vi "Global Mapper H.vi"(0 "GIC Input":T1={"     Use ?\nOff       On"=[FALSE, TRUE, FALSE, TRUE], "Mode:"=FALSE, "WP Data"="", "Hokuyo Port"="COM7", "Prop  Port"="COM6", "Compass Port"="", "GPS Port"="", "Num of WPs"=0, "WP Lats and Longs"={"WP Lats"=[], "WP Longs"=[]}, "Obst Lats and Longs"={"Obst Lats"=[], "Obst Longs"=[]}, "Parameters"=[], "GPS Data"=[], "Compass"=0.0, "LMS Vector"=[], "Vision Vector"=[], "Direction Cmd"=0.0, "Speed Cmd"=0.0, "WP Vector"=[], "WP Number"=0, "Extra"=0, "SW Map"=[], "Path Cluster"={"Path x node"=[], "Path y node"=[]}, "Sim Course"=[]} {"Obst Lats and Longs"."Obst Longs" format="%#_8g"; "Obst Lats and Longs"."Obst Lats" format="%#_8g"}, 3 "sim path":path) -> (9 "picture out":picture)   [LabVIEW 2014]
panel:
  # "Global Mapper H"
  # "Inputs:"
  # "Output:"
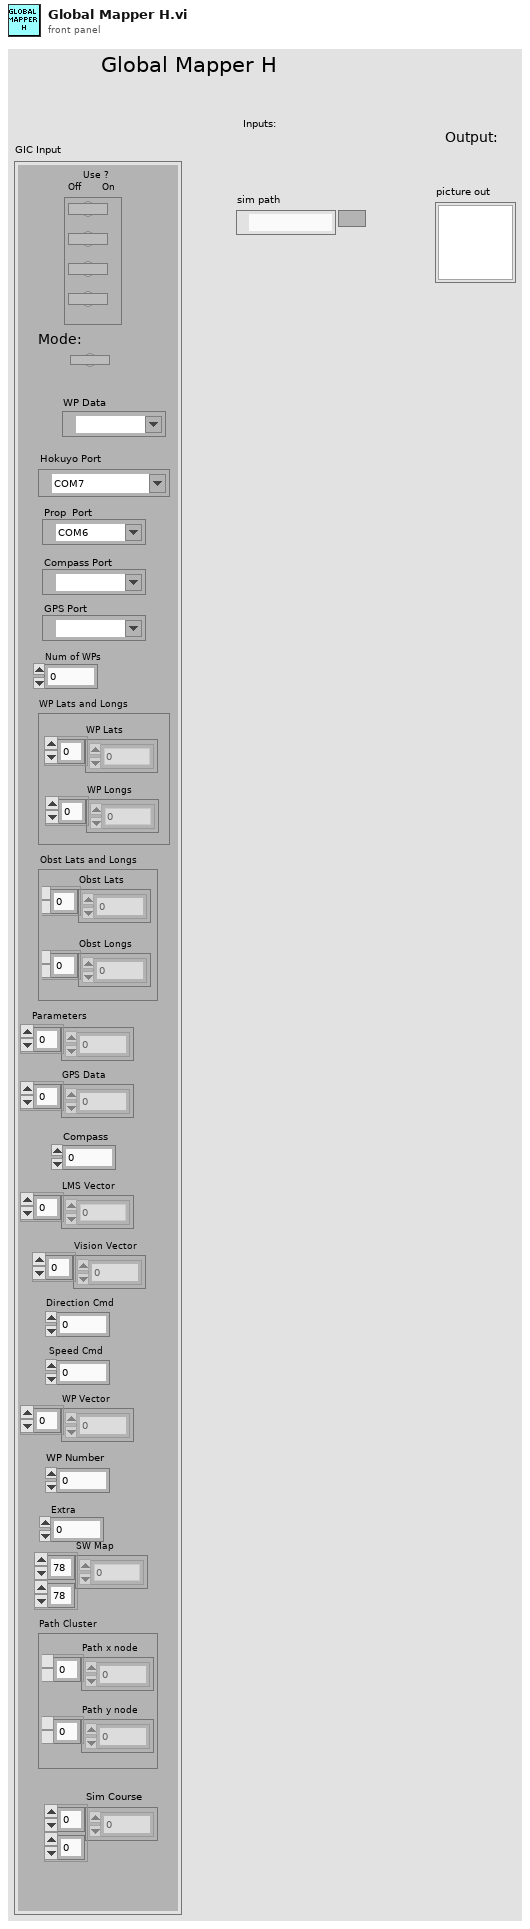
[diagram p1: front panel]
types:
  T1 = cluster{"     Use ?\nOff       On":bool[], "Mode:":bool, "WP Data":refnum<visa-resource-name>, "Hokuyo Port":refnum<visa-resource-name>, "Prop  Port":refnum<visa-resource-name>, "Compass Port":refnum<visa-resource-name>, "GPS Port":refnum<visa-resource-name>, "Num of WPs":i16, "WP Lats and Longs":cluster{"WP Lats":dbl[], "WP Longs":dbl[]}, "Obst Lats and Longs":cluster{"Obst Lats":dbl[], "Obst Longs":dbl[]}, "Parameters":dbl[], "GPS Data":dbl[], "Compass":dbl, "LMS Vector":dbl[], "Vision Vector":dbl[], "Direction Cmd":dbl, "Speed Cmd":dbl, "WP Vector":dbl[], "WP Number":i32, "Extra":i16, "SW Map":i32[][], "Path Cluster":cluster{"Path x node":dbl[], "Path y node":dbl[]}, "Sim Course":i8[][]}
  T2 = typedef "imagedata.ctl" = cluster{"image type":i32, "image depth":i32, "image":u8[], "mask":u8[], "colors":u32[], "Rectangle":cluster{"left":i16, "top":i16, "right":i16, "bottom":i16}}
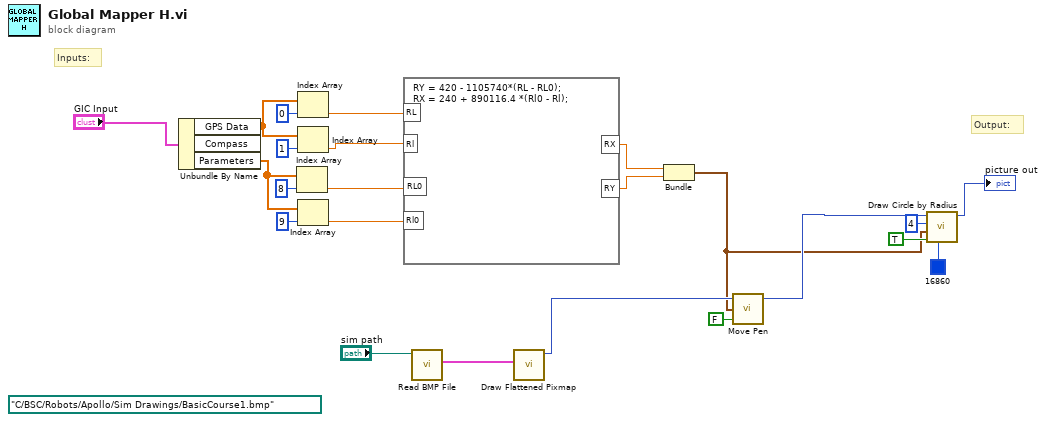
[diagram p0: block diagram]
diagram:
  (unwired) path "C:/BSC/Robots/Apollo/Sim Drawings/BasicCourse1.bmp" ("path to BMP file")
  # "Output:"
  # "Inputs:"
  n1 = Unbundle By Name("GIC Input") -> ("GPS Data"=w20:dbl[], "Parameters"=w15:dbl[])  [unwired: 1 out]
  n2 = Index Array(array=w15, index=8) -> (element=w17:dbl)
  n3 = Index Array(array=w20, index=0) -> (element=w22:dbl)
  n4 = Index Array(array=w20, index=1) -> (element=w18:dbl)
  n5 = Index Array(array=w15, index=9) -> (element=w13:dbl)
  n6 = formula code="RY = 420 - 1105740*(RL - RL0);\nRX = 240 + 890116.4 *(Rl0 - Rl);"("RL"=w22, "Rl"=w18, "RL0"=w17, "Rl0"=w13) -> ("RY"=w9:dbl, "RX"=w10:dbl)
  n7 = call <vilib>:"Read BMP File.vi"("path to BMP file"="sim path") -> ("image data"=w12:T2)  [unwired: 8 in, 2 out]
  n8 = call <vilib>:"Draw Flattened Pixmap.vi"("image data"=w12) -> ("new picture"=w8:picture)  [unwired: 8 in]
  n9 = Bundle("RX"=w10, "RY"=w9) -> (w3:cluster{"RX":dbl, "RY":dbl})  [unwired: 1 in]
  n10 = call <vilib>:"Move Pen.vi"("absolute coordinates?(T)"=FALSE, "new position"=w3, "picture"=w8) -> ("new picture"=w4:picture)  [unwired: 2 in]
  n11 = call <vilib>:"Draw Circle by Radius.vi"("color(black)"=u32 16860, "fill?(F)"=TRUE, "pixel center"=w3, "radius"=i16 4, "picture"=w4) -> ("new picture"=→"picture out":picture)  [unwired: 6 in]
